vi "Programmatic Build Command Line Target.vi"() -> ()   [LabVIEW 2019]
doc: "The VI is called from the command line based on a command line string generated by Passing Command Line Parameters.vi."
uses:
  <vilib>/AppBuilder/AB_API_Simple/Build (path).vi
  <vilib>/AppBuilder/AB_API_Simple/NI_App_Builder_API.lvlib
panel:
  out "Generated Files from Build":path[](array[path])
  out "Command Line Arguments":string[](array[string])
  # "When calling this VI from the command line, the parameters for calling the Application Builder API will be used. The Command Line Arguments array displays the arguments retrieved from the Application:Command Line Arguments property.\n\nNote: This VI must be set to Run when opened in order to retrieve the command line parameters properly. Go to File > VI Properties > Execution to set this property."
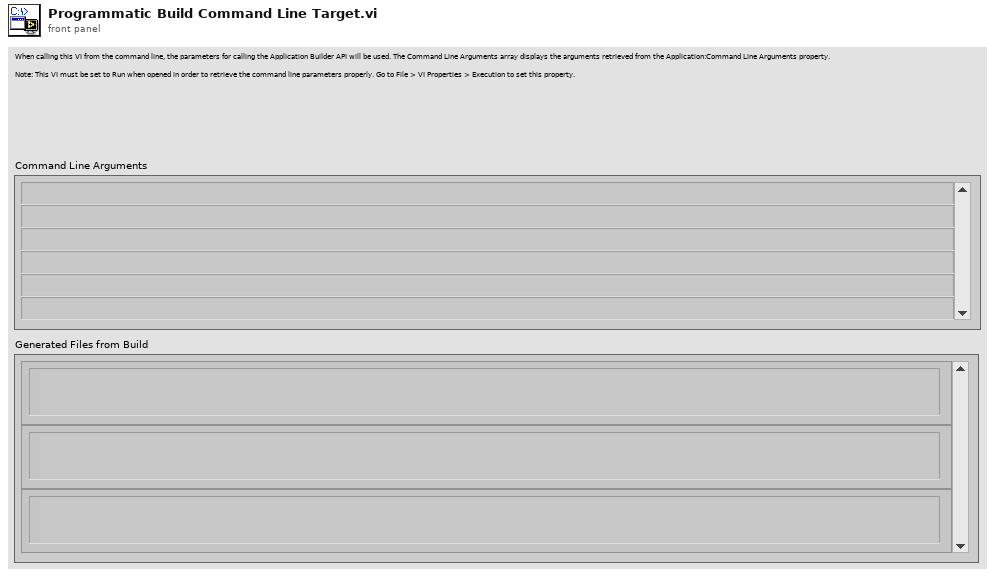
[diagram p1: front panel]
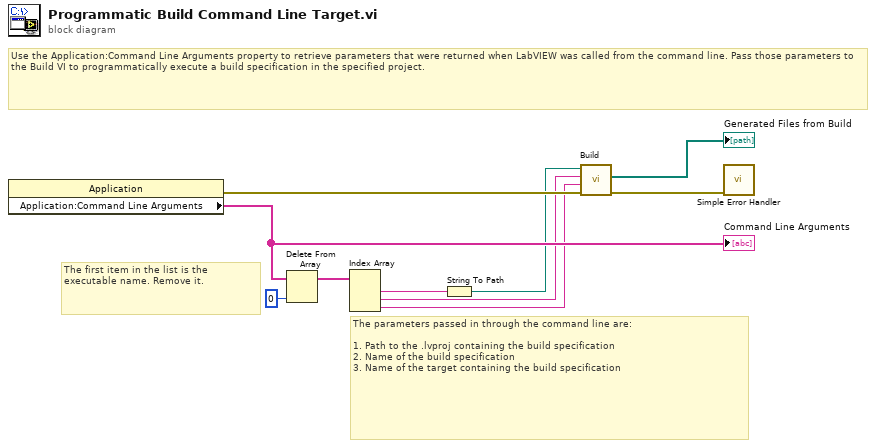
[diagram p0: block diagram]
diagram:
  # "The parameters passed in through the command line are:\n\n1. Path to the .lvproj containing the build specification\n2. Name of the build specification\n3. Name of the target containing the build specification"
  # "Use the Application:Command Line Arguments property to retrieve parameters that were returned when LabVIEW was called from the command line. Pass those parameters to the Build VI to programmatically execute a build specification in the specified project."
  # "The first item in the list is the executable name. Remove it."
  n1 = property class="Application"() -> (error out=w7:errorcluster, "Application:Command Line Arguments"=w10:string[])  [unwired: 2 in, 1 out]
  "Command Line Arguments" <- w10
  n2 = Delete From Array(array=w10, index=0 ("length")) -> (array with subset deleted=w8:string[])  [unwired: 1 in, 1 out]
  n3 = Index Array(array=w8) -> (element #1=w2:string, element #2=w4:string, element #3=w3:string)  [unwired: 3 in]
  n4 = String To Path(string=w2) -> (path=w1:path)
  n5 = call-poly <vilib>:"Build.vi"("error in (no error)"=w7, "Name of target (My Computer)"=w3, "Name of build specification (if empty: build all)"=w4, "Path to project"=w1) -> ("error out"=w6:errorcluster, "Generated files"=→"Generated Files from Build":path[])  [unwired: 6 in]
  n6 = call <vilib>:"Simple Error Handler.vi"("error in (no error)"=w6) -> ()  [unwired: 1 in, 8 out]
